vi "Configuration Manager.vi"(7 "Actions":T4, 10 "Owner":string, 11 "Mutex Name":string) -> (3 "Success?":bool)   [LabVIEW 2021]
uses:
  <vilib>/myRIO/Common/Instrument Driver Framework/Utilities/typedefs/Resource Manager Action Enum.ctl
  <vilib>/myRIO/Common/Instrument Driver Framework/Utilities/typedefs/Mutex Collection.ctl
  <vilib>/myRIO/Common/Instrument Driver Framework/Utilities/typedefs/Named Mutex.ctl
  <vilib>/myRIO/Common/Instrument Driver Framework/Utilities/typedefs/Reentrant Mutex.ctl
panel:
  out "Mutex Collection":T1
  out "error out":errorcluster
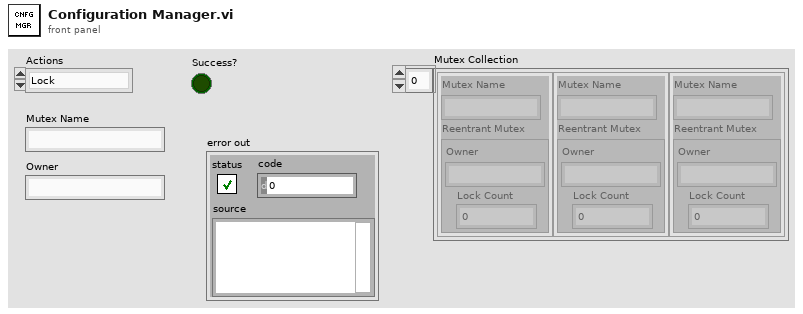
[diagram p1: front panel]
types:
  T1 = typedef "Mutex Collection.ctl" = T2[]
  T2 = typedef "Named Mutex.ctl" = cluster{"Mutex Name":string, "Reentrant Mutex":T3}
  T3 = typedef "Reentrant Mutex.ctl" = cluster{"Owner":string, "Lock Count":u32}
  T4 = typedef "Resource Manager Action Enum.ctl" = enum16{"Lock", "Unlock"}
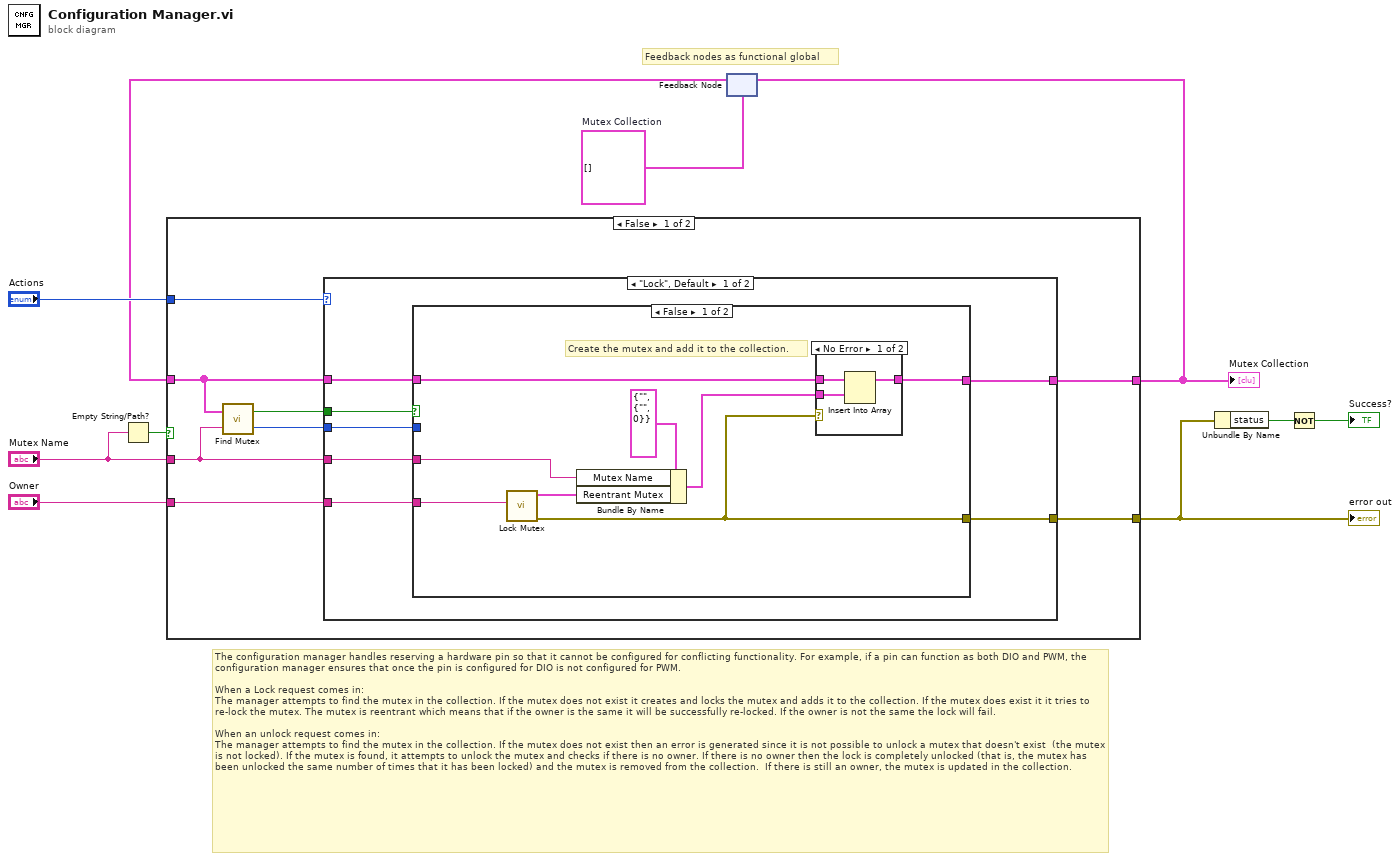
[diagram p0: block diagram]
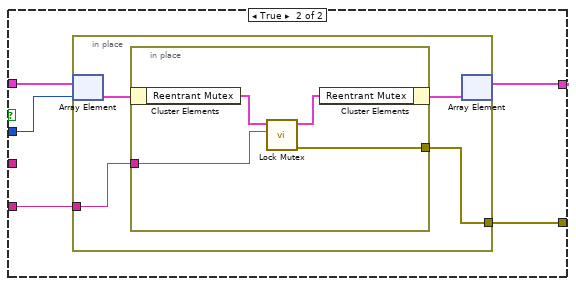
[diagram p3: hidden frame]
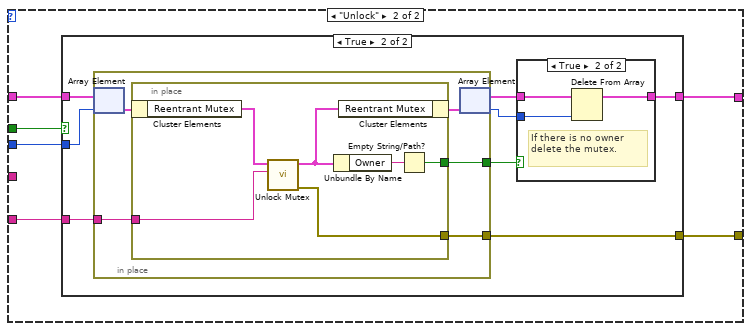
[diagram p4: hidden frame]
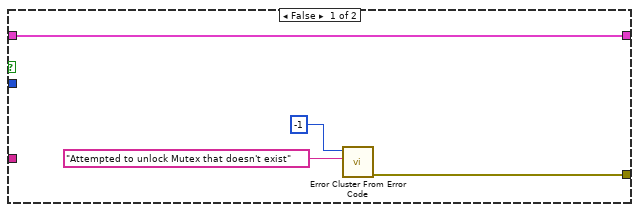
[diagram p5: hidden frame]
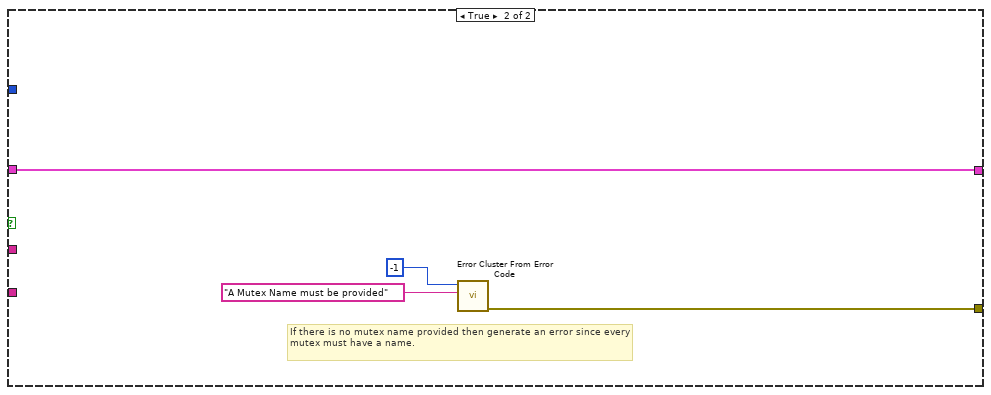
[diagram p7: hidden frame]
diagram:
  w4 = T1 []  # Mutex Collection
  # "The configuration manager handles reserving a hardware pin so that it cannot be configured for conflicting functionality. For example, if a pin can function as both DIO and PWM, the configuration manager ensures that once the pin is configured for DIO is not configured for PWM.\n\nWhen a Lock request comes in:\nThe manager attempts to find the mutex in the collection. If the mutex does not exist it creates and locks the mutex and adds it to the collection. If the mutex does exist it it tries to re-lock the mutex. The mutex is reentrant which means that if the owner is the same it will be successfully re-locked. If the owner is not the same the lock will fail.\n\nWhen an unlock request comes in:\nThe manager attempts to find the mutex in the collection. If the mutex does not exist then an error is generated since it is not possible to unlock a mutex that doesn't exist  (the mutex is not locked). If the mutex is found, it attempts to unlock the mutex and checks if there is no owner. If there is no owner then the lock is completely unlocked (that is, the mutex has been unlocked the same number of times that it has been locked) and the mutex is removed from the collection.  If there is still an owner, the mutex is updated in the collection."
  # "Feedback nodes as functional global"
  n1 = Empty String/Path?(string/path="Mutex Name") -> (empty?=w2:bool)
  n2 = feedback #1(w4) -> (w3:T1)
  n3 = case shown="False" w2 {
    tunnel: "Actions" -> [w18 _]
    tunnel: "Owner" -> [w17 _]
    tunnel: [w16 w87] -> w8
    tunnel: [w15 w84] -> w5
    tunnel: w3 -> [w13 w84]
    tunnel: "Mutex Name" -> [w11 _]
    frame False {
      n4 = call <vilib>:"Find Mutex.vi"("Mutex Name"=w11, "Mutex Collection"=w13) -> ("Index"=w12:i32, "Found?"=w14:bool)
      n5 = case shown="\"Lock\", Default" w18 {
        tunnel: w11 -> [w21 _]
        tunnel: w13 -> [w25 w55]
        tunnel: w17 -> [w24 w52]
        tunnel: [w23 w51] -> w16
        tunnel: [w22 w53] -> w15
        tunnel: w14 -> [w20 w56]
        tunnel: w12 -> [w19 w54]
        frame "Lock", Default {
          n6 = case shown="False" w20 {
            tunnel: w25 -> [w29 w41]
            tunnel: w19 -> [_ w42]
            tunnel: w24 -> [w33 w40]
            tunnel: [w26 w39] -> w23
            tunnel: [w28 w38] -> w22
            tunnel: w21 -> [w30 _]
            frame False {
              # "Create the mutex and add it to the collection."
              n7 = call <vilib>:"Lock Mutex.vi"("Owner"=w33) -> ("error out"=w26:errorcluster, "Mutex Out"=w32:T3)  [unwired: 9 in]
              n8 = Bundle By Name(cluster=T2 {"Mutex Name"="", "Reentrant Mutex"={"Owner"="", "Lock Count"=0}} ("Named Mutex"), "Mutex Name"=w30, "Reentrant Mutex"=w32) -> (w27:T2)
              n9 = case shown="No Error" w26 {
                tunnel: w29 -> [w36 w37]
                tunnel: [w35 w37] -> w28
                tunnel: w27 -> [w34 _]
                frame No Error {
                  n10 = Insert Into Array(array=w36, new element=w34) -> (w35:T1)  [unwired: 1 in]
                }
                frame Error {
                }
              }
            }
            frame True {
              n11 = in-place {
                in-place-border: w40 -> [w46]
                in-place-border: [w45] -> w39
                n12 = in-place-array #2(w41, w42) -> (w44:T2)
                n13 = in-place {
                  in-place-border: w46 -> [w50]
                  in-place-border: [w49] -> w45
                  n14 = in-place-cluster #3(w44) -> ("Reentrant Mutex"=w48:T3)
                  n15 = call <vilib>:"Lock Mutex.vi"("Owner"=w50, "Mutex In"=w48) -> ("error out"=w49:errorcluster, "Mutex Out"=w47:T3)  [unwired: 8 in]
                  n16 = in-place-cluster #3("Reentrant Mutex"=w47) -> (w43:T2)
                }
                n17 = in-place-array #2(w43) -> (w38:T1)  [unwired: 1 out]
              }
            }
          }
        }
        frame "Unlock" {
          n18 = case shown="True" w56 {
            tunnel: w55 -> [w57 w66]
            tunnel: w54 -> [_ w65]
            tunnel: [w57 w67] -> w53
            tunnel: w52 -> [_ w64]
            tunnel: [w60 w61] -> w51
            frame False {
              n19 = call <vilib>:"Error Cluster From Error Code.vi"("error message (\"\")"="Attempted to unlock Mutex that doesn't exist" ("error message (\"\")"), "error code (0)"=-1) -> ("error out"=w60:errorcluster)  [unwired: 7 in]
            }
            frame True {
              n20 = in-place {
                in-place-border: [w73] -> w68
                in-place-border: w64 -> [w71]
                in-place-border: [w69] -> w61
                n21 = in-place-array #4(w66, w65) -> (w72:T2)
                n22 = in-place {
                  in-place-border: [w78] -> w73
                  in-place-border: w71 -> [w75]
                  in-place-border: [w74] -> w69
                  n23 = in-place-cluster #5(w72) -> ("Reentrant Mutex"=w77:T3)
                  n24 = call <vilib>:"Unlock Mutex.vi"("Owner"=w75, "Mutex In"=w77) -> ("error out"=w74:errorcluster, "Mutex Out"=w76:T3)  [unwired: 8 in]
                  n25 = Unbundle By Name(w76) -> ("Owner"=w79:string)
                  n26 = in-place-cluster #5("Reentrant Mutex"=w76) -> (w70:T2)
                  n27 = Empty String/Path?(string/path=w79) -> (empty?=w78:bool)
                }
                n28 = in-place-array #4(w70) -> (w63:T1, w62:i32)
              }
              n29 = case shown="True" w68 {
                tunnel: w63 -> [w80 w83]
                tunnel: w62 -> [_ w82]
                tunnel: [w80 w81] -> w67
                frame False {
                }
                frame True {
                  # "If there is no owner delete the mutex."
                  n30 = Delete From Array(array=w83, index=w82) -> (array with subset deleted=w81:T1)  [unwired: 1 in, 1 out]
                }
              }
            }
          }
        }
      }
    }
    frame True {
      # "If there is no mutex name provided then generate an error since every mutex must have a name."
      n31 = call <vilib>:"Error Cluster From Error Code.vi"("error message (\"\")"="A Mutex Name must be provided" ("error message (\"\")"), "error code (0)"=-1) -> ("error out"=w87:errorcluster)  [unwired: 7 in]
    }
  }
  "error out" <- w8
  "Mutex Collection" <- w5
  n32 = feedback-in #1(w5) -> ()
  n33 = Unbundle By Name(w8) -> ("status"=w7:bool)
  n34 = Not(x=w7) -> (.not. x?=→"Success?":bool)
